vi "Configure OSC CRANge Scale query.vi"(8 "error in (no error)":errorcluster, 9 "range":enum16{"MIN", "NOW", "MAX"}(ring)=enum."NOW", 10 "Step":T1=1 min=1 max=99 step=1, 11 "VISA resource in":refnum<visa-resource-name>) -> (0 "error out":errorcluster, 2 "Scale range":string, 3 "VISA resource out":refnum<visa-resource-name>)   [LabVIEW 2025, in "Chroma 19052.lvlib"]
uses:
  <instrlib>/Chroma 19052/Chroma 19052.lvlib
  <instrlib>/Chroma 19052/Public/Utility/Type Def/steps--numeric.ctl
panel:
  # "Query OSC Capacitance RANGE"
  # "Scale          Ranges\n    1          0.001 - 9.999nF\n    2            0.01 - 99.99nF   \n    3             0.1 - 500nF"
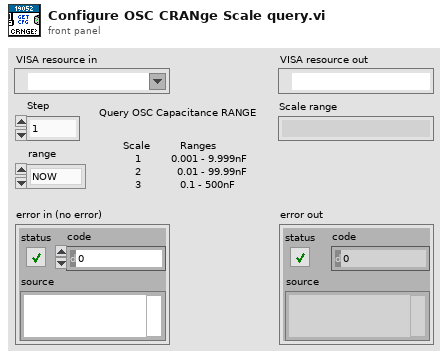
[diagram p1: front panel]
types:
  T1 = typedef "Chroma 19052.lvlib/steps--numeric.ctl" = u8
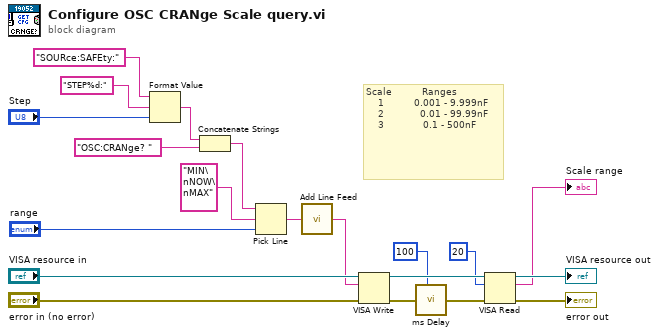
[diagram p0: block diagram]
diagram:
  # "Scale          Ranges\n    1          0.001 - 9.999nF\n    2            0.01 - 99.99nF   \n    3             0.1 - 500nF"
  n1 = Format Value(string ("")="SOURce:SAFEty:", format string="STEP%d:", value (0)="Step") -> (output string=w11:string)
  n2 = Concatenate Strings(w11, "OSC:CRANge? ") -> (w9:string)
  n3 = Pick Line(string ("")=w9, multi-line string="MIN\nNOW\nMAX", line index="range") -> (output string=w2:string)
  n4 = call <instrlib>:"Add Line Feed.vi"("Command string"=w2) -> ("Concatenated string"=w1:string)  [unwired: 4 in]
  n5 = VISA Write(VISA resource name="VISA resource in", write buffer=w1, error in (no error)="error in (no error)") -> (VISA resource name out=w7:refnum<visa-resource-name>, error out=w5:errorcluster)  [unwired: 1 out]
  n6 = call <instrlib>:"ms Delay.vi"("miliseconds to wait"=u32 100, "error in (no error)"=w5) -> ("error out"=w4:errorcluster)  [unwired: 6 in, 1 out]
  n7 = VISA Read(VISA resource name=w7, byte count=u32 20, error in (no error)=w4) -> (VISA resource name out=→"VISA resource out":refnum<visa-resource-name>, read buffer=→"Scale range":string, error out=→"error out":errorcluster)  [unwired: 1 out]
